vi "SelectMenu3.vi"(6 "Click Type":T1, 7 "Id":string, 8 "Point":T3, 9 "Item Index":u32, 10 "XRef":refnum<vi>, 11 "State In":T2={"Output Type"=variant(dbl 0.0), "Typedef Name"="", "Input Type"=variant, "Constant Types"=[], "Error"={"status"=FALSE, "code"=0, "source"=""}, "Typedef Path"=path "", "Names"=[], "Event Cluster Name"=""}) -> (0 "Reply":string[](array[string]), 3 "State Out":T2={"Output Type"=variant(dbl 0.0), "Typedef Name"="", "Input Type"=variant, "Constant Types"=[], "Error"={"status"=FALSE, "code"=0, "source"=""}, "Typedef Path"=path "", "Names"=[], "Event Cluster Name"=""})   [LabVIEW 2015, in "Create-Signals.xnode"]
doc: "This ability VI is called after the user selects an item from a portion of the menu defined during BuildMenu. Click Type is the type of click that led to the building of the menu whose selection is being handled by this VI. ItemIndex is the index of the element in the array used when you specified the popup menu. Id is the id you associated with the item in BuildMenu3. Point is the location where the user clicked to build the menu relative to the top-left corner of the XNode. You can display a dialog in response to a user selection if you wish. Use Reply to inform LabVIEW of any actions it needs to take.\n\nDefault behavior: None.\n\nThis ability provides UI and OS messages are handled.\n\nSee also: BuildMenu3"
uses:
  Create-Signals.xnode
  State.ctl
  <vilib>/XNodeSupport/XNodePoint.ctl
  <vilib>/XNodeSupport/XNodeInt.ctl
  <vilib>/XNodeSupport/XNodeClickTypes.ctl
  <vilib>/XNodeSupport/NI_XNodeSupport.lvlib
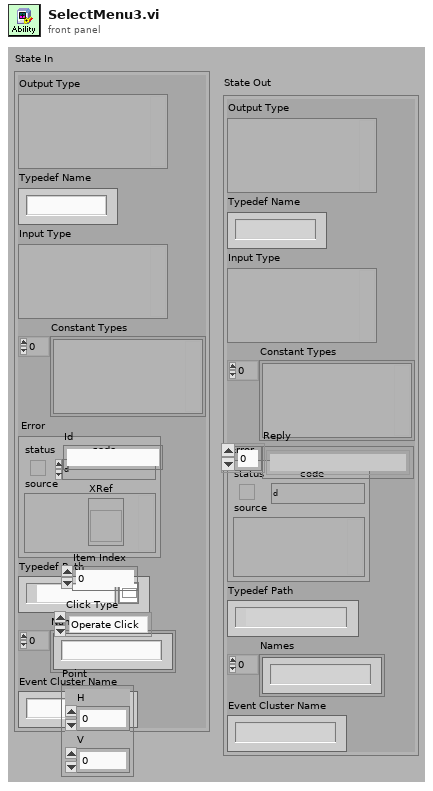
[diagram p1: front panel]
types:
  T1 = typedef "NI_XNodeSupport.lvlib/XNodeClickTypes.ctl" = enum32{"Operate Click", "Popup Click"}
  T2 = typedef "Create-Signals.xnode/State.ctl" = cluster{"Output Type":variant, "Typedef Name":string, "Input Type":variant, "Constant Types":variant[], "Error":errorcluster, "Typedef Path":path, "Names":string[], "Event Cluster Name":string}
  T3 = typedef "NI_XNodeSupport.lvlib/XNodePoint.ctl" = cluster{"H":T4, "V":T4}
  T4 = typedef "NI_XNodeSupport.lvlib/XNodeInt.ctl" = i32
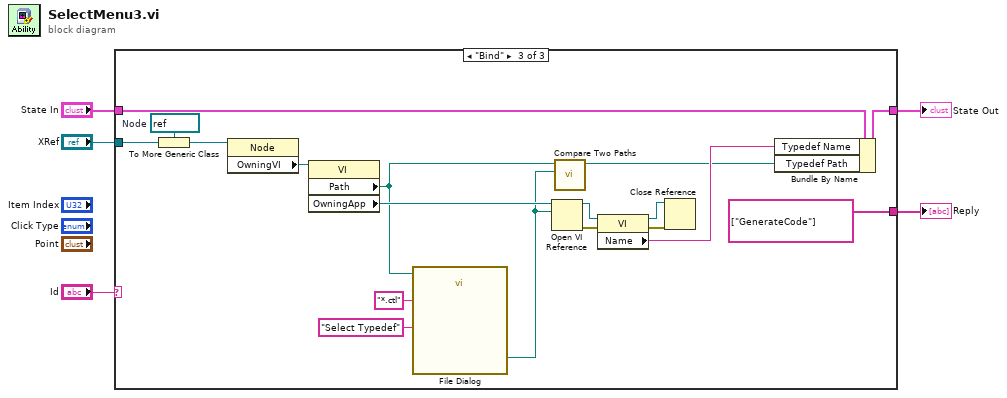
[diagram p0: block diagram]
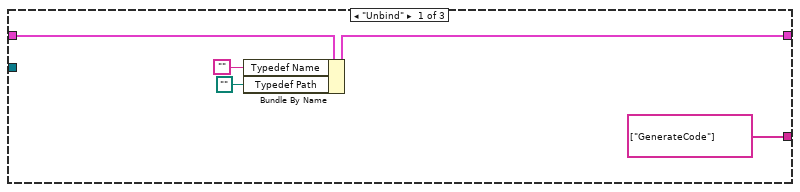
[diagram p2: hidden frame]
diagram:
  n1 = case shown="\"Bind\"" "Id" {
    tunnel: [w9 w11 w28] -> w4
    tunnel: "State In" -> [w10 w11 w29]
    tunnel: "XRef" -> [_ _ w27]
    tunnel: [string[] ["GenerateCode"] ("Reply") _ string[] ["GenerateCode"] ("Reply")] -> w1
    frame "Unbind" {
      n2 = Bundle By Name(cluster=w10, "Typedef Name"="", "Typedef Path"=path "") -> (w9:T2)
    }
    frame Default {
    }
    frame "Bind" {
      w26 = refnum<vi> refnum  # Node
      n3 = To More Generic Class(target class=w26, reference=w27) -> (generic class reference=w25:refnum<vi>)
      n4 = property class="Node"(reference=w25) -> ("OwningVI"=w24:refnum<vi>)  [unwired: 1 in, 2 out]
      n5 = property class="VI"(reference=w24) -> ("Path"=w14:path, "OwningApp"=w20:refnum<vi>)  [unwired: 1 in, 2 out]
      n6 = call "File Dialog"("start path"=w14, "prompt"="Select Typedef", "pattern (all files)"="*.ctl") -> ("selected path"=w13:path)  [unwired: 9 in, 3 out]
      n7 = Open VI Reference(application reference (local)=w20, vi path=w13) -> (vi reference=w17:refnum<vi>, error out=w19:errorcluster)  [unwired: 4 in]
      n8 = call <vilib>:"Compare Two Paths.vi"("Path 2"=w13, "Path 1"=w14) -> ("Relative Path from 1 to 2"=w12:path)  [unwired: 6 in, 3 out]
      n9 = property class="VI"(reference=w17, error in=w19) -> (reference out=w16:refnum<vi>, error out=w18:errorcluster, "Name"=w15:string)
      n10 = Close Reference(reference=w16, error in (no error)=w18) -> ()  [unwired: 1 out]
      n11 = Bundle By Name(cluster=w29, "Typedef Name"=w15, "Typedef Path"=w12) -> (w28:T2)
    }
  }
  "State Out" <- w4
  "Reply" <- w1
